vi "HW_Send_Command.vi"(3 "Error In":errorcluster, 4 "HW Command":T3, 5 "Port info in":T2={"Type"=enum."Serial (VISA)", "Serial Port"="", "IP Address"="0.0.0.0"}) -> (0 "Error Out":errorcluster, 1 "Message":string, 2 "Port info out":T2={"Type"=enum."Serial (VISA)", "Serial Port"="", "IP Address"="0.0.0.0"})   [LabVIEW 2018, in "HW Interaction.lvlib"]
uses:
  HW Interaction.lvlib
  Public API/Typedefs/CTL_Port_connection_type.ctl
  Typedefs/CTL_HW_Interaction_Commands.ctl
  <vilib>/Instr/_visa.llb/VISA Flush IO Buffer Mask.ctl
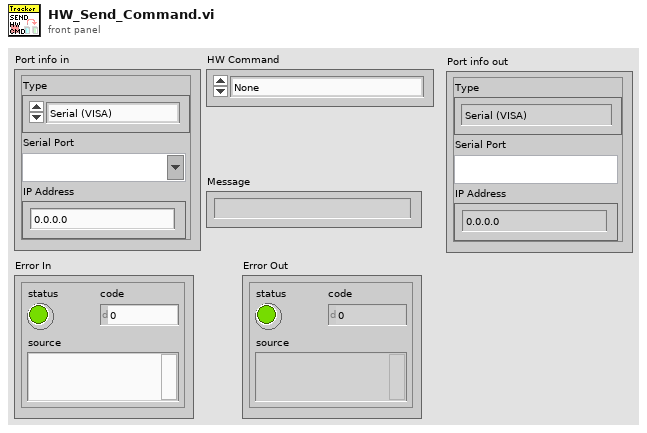
[diagram p1: front panel]
types:
  T1 = typedef "HW Interaction.lvlib/CTL_Port_connection_type.ctl" = enum16{"Serial (VISA)", "TCP/IP"}
  T2 = cluster{"Type":T1, "Serial Port":refnum<visa-resource-name>, "IP Address":string}
  T3 = typedef "HW Interaction.lvlib/CTL_HW_Interaction_Commands.ctl" = enum16{"None", "Acquisition Stop", "Connection Stop and Close"}
  T4 = typedef "VISA Flush IO Buffer Mask.ctl" = u16
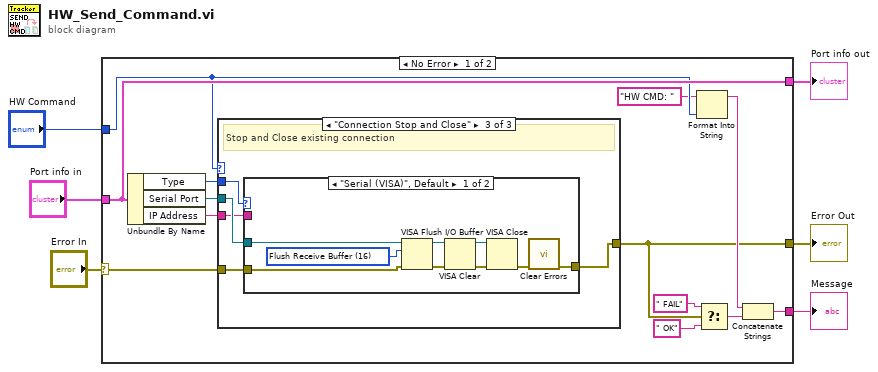
[diagram p0: block diagram]
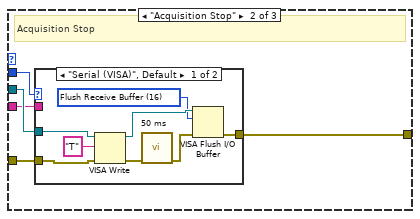
[diagram p3: hidden frame]
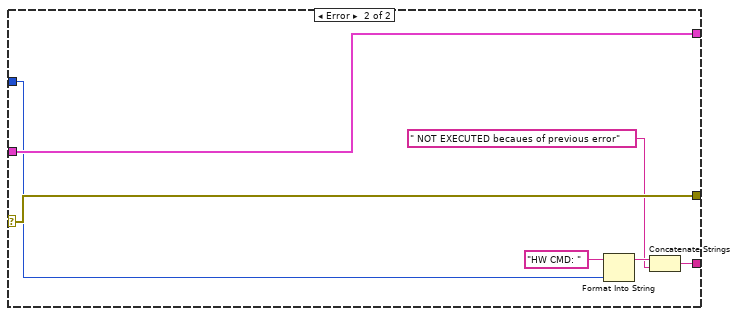
[diagram p6: hidden frame]
diagram:
  n1 = case shown="No Error" "Error In" {
    selector: "Error In" -> [w19 w55]
    tunnel: "Port info in" -> [w15 w56]
    tunnel: "HW Command" -> [w14 w53]
    tunnel: [w15 w56] -> w3
    tunnel: [w7 w55] -> w2
    tunnel: [w8 w51] -> w1
    frame No Error {
      n2 = Unbundle By Name(w15) -> ("Type"=w18:T1, "Serial Port"=w17:refnum<visa-resource-name>, "IP Address"=w16:string)
      n3 = case shown="\"Connection Stop and Close\"" w14 {
        tunnel: [w20 w25 w39] -> w7
        tunnel: w19 -> [w20 w24 w38]
        tunnel: w18 -> [_ w23 w37]
        tunnel: w17 -> [_ w22 w36]
        tunnel: w16 -> [_ w21 w35]
        frame "None", Default {
          # "Nothing happens here"
        }
        frame "Acquisition Stop" {
          # "Acquisition Stop"
          n4 = case shown="\"Serial (VISA)\", Default" w23 {
            tunnel: [w31 w34] -> w25
            tunnel: w24 -> [w30 w34]
            tunnel: w22 -> [w26 _]
            tunnel: w21 -> [_ _]
            frame "Serial (VISA)", Default {
              w28 = T4 16 items=["Flush Receive Buffer"=16, "Write Transmit Buffer to Device"=32, "Flush Receive Buffer (No I/O)"=64, "Flush Transmit Buffer"=128] ("Mask")
              n5 = VISA Write(VISA resource name=w26, write buffer="T", error in (no error)=w30) -> (VISA resource name out=w32:refnum<visa-resource-name>, error out=w33:errorcluster)  [unwired: 1 out]
              n6 = call "50 ms"("error in (no error)"=w33) -> ("error out"=w27:errorcluster)  [unwired: 10 in]
              n7 = VISA Flush I/O Buffer(VISA resource name=w32, mask (16)=w28, error in (no error)=w27) -> (error out=w31:errorcluster)  [unwired: 1 out]
            }
            frame "TCP/IP" {
            }
          }
        }
        frame "Connection Stop and Close" {
          # "Stop and Close existing connection"
          n8 = case shown="\"Serial (VISA)\", Default" w37 {
            tunnel: [w41 w49] -> w39
            tunnel: w38 -> [w47 w49]
            tunnel: w36 -> [w46 _]
            tunnel: w35 -> [_ _]
            frame "Serial (VISA)", Default {
              w48 = T4 16 items=["Flush Receive Buffer"=16, "Write Transmit Buffer to Device"=32, "Flush Receive Buffer (No I/O)"=64, "Flush Transmit Buffer"=128] ("Mask")
              n9 = VISA Flush I/O Buffer(VISA resource name=w46, mask (16)=w48, error in (no error)=w47) -> (VISA resource name out=w40:refnum<visa-resource-name>, error out=w42:errorcluster)
              n10 = VISA Clear(VISA resource name=w40, error in (no error)=w42) -> (VISA resource name out=w44:refnum<visa-resource-name>, error out=w43:errorcluster)
              n11 = VISA Close(VISA resource name=w44, error in (no error)=w43) -> (error out=w45:errorcluster)
              n12 = call <vilib>:"Clear Errors.vi"("error in (no error)"=w45) -> ("error out"=w41:errorcluster)  [unwired: 5 in, 1 out]
            }
            frame "TCP/IP" {
            }
          }
        }
      }
      n13 = Format Into String(initial string="HW CMD: ", w14) -> (resulting string=w12:string)  [unwired: 2 in, 1 out]
      n14 = Select(t=" FAIL", s=w7, f=" OK") -> (s? t:f=w9:string)
      n15 = Concatenate Strings(w12, w9) -> (w8:string)
    }
    frame Error {
      n16 = Format Into String(initial string="HW CMD: ", w53) -> (resulting string=w52:string)  [unwired: 2 in, 1 out]
      n17 = Concatenate Strings(w52, " NOT EXECUTED becaues of previous error" ("string")) -> (w51:string)
    }
  }
  "Error Out" <- w2
  "Port info out" <- w3
  "Message" <- w1
